vi "Ch Get FPDIV.vi"(7 "DIV":u16, 9 "FP":u16, 10 "Channel":u8, 11 "devId":i32) -> (1 "FP out":u16, 2 "devId out":i32, 3 "function return":i32, 5 "DIV out":u16)   [LabVIEW 2013, in "CHR34XXX.lvlib"]
doc: "DLL BOOL __stdcall CHR34XXX_Ch_GetFPDIV(IN int devId,IN BYTE Channel,IN WORD *FP,IN WORD *DIV);"
uses:
  CHR34XXX.lvlib
  CHR34XXX.dll
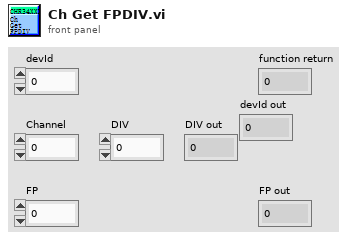
[diagram p1: front panel]
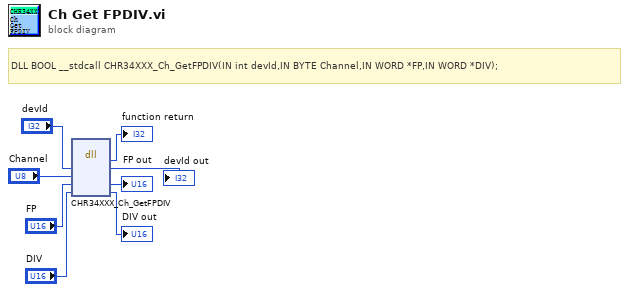
[diagram p0: block diagram]
diagram:
  # "DLL BOOL __stdcall CHR34XXX_Ch_GetFPDIV(IN int devId,IN BYTE Channel,IN WORD *FP,IN WORD *DIV);"
  n1 = dll-call lib="C:/Users/Administrator/Desktop/CHR34XXX_lv/lv_lib/CHR34XXX.*" fn="CHR34XXX_Ch_GetFPDIV"("devId"="devId", "Channel"="Channel", "FP"="FP", "DIV"="DIV") -> (→"function return":i32, "devId"=→"devId out":i32, "FP"=→"FP out":u16, "DIV"=→"DIV out":u16)  [unwired: 4 in, 2 out]
